vi "List Files.vi"(1 "File Pattern[] (e.g. *.vi)":string[](array[string]), 2 "Root Path":path) -> (0 "File Path[]":path[](array[path]))   [LabVIEW 2017, in "DocTools.lvlib"]
uses:
  DocTools.lvlib
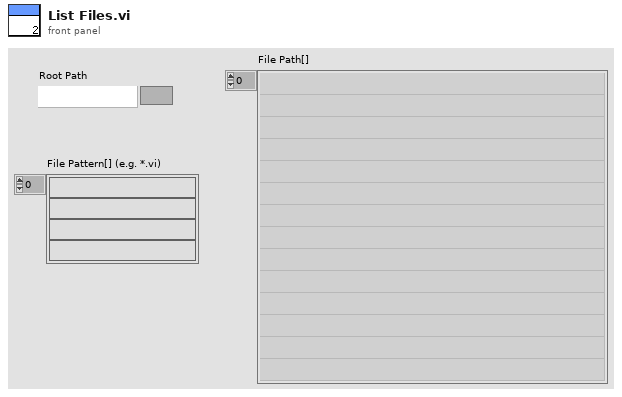
[diagram p1: front panel]
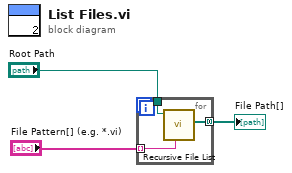
[diagram p0: block diagram]
diagram:
  n1 = for {
    tunnel: "File Pattern[] (e.g. *.vi)" -> [w6] mode=indexing
    tunnel: [w5] -> w2 mode=concatenating
    tunnel: "Root Path" -> [w4]
    n2 = call <vilib>:"Recursive File List.vi"("pattern"=w6, "Folder Path"=w4) -> ("All Files in Dir"=w5:path[])  [unwired: 5 in, 4 out]
  }
  "File Path[]" <- w2
